vi "State_Machine.vi"(8 "error in (no error)":errorcluster caption="entrée d'erreur (pas d'erreur)", 11 "Get_Voltage en entrée":refnum<class "Zigbee_Send_Msg_Default.lvclass">) -> (0 "error out":errorcluster caption="sortie d'erreur", 2 "Json_String":string, 3 "Get_Voltage en sortie":refnum<class "Zigbee_Send_Msg_Default.lvclass">)   [LabVIEW 2020, in "Library Test.lvlib" / "Zigbee_Send_Msg_Default.lvclass"]
uses:
  Zigbee_Send_Msg_Default.lvclass
  C:/Users/ngarcin/OneDrive - Altyor/Standard TB/Class/Test/Zigbee_Send_Msg/Zigbee_Send_Msg.lvclass
  Zigbee_Send_Msg/Zigbee_Send_Msg.lvclass
  Zigbee_Send_Msg_Default.lvclass/Zigbee_Send_Msg_Default.ctl
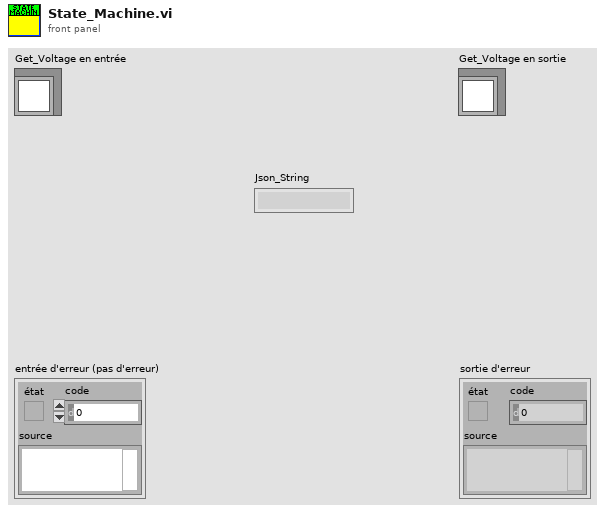
[diagram p1: front panel]
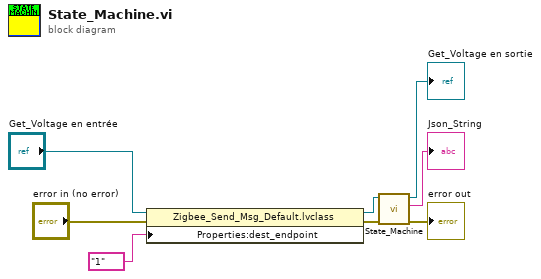
[diagram p0: block diagram]
diagram:
  n1 = property class="Zigbee_Send_Msg_Default.lvclass"(reference="Get_Voltage en entrée", error in="error in (no error)", "Properties:dest_endpoint"="1") -> (reference out=w4:refnum<class "Zigbee_Send_Msg_Default.lvclass">, error out=w1:errorcluster)
  n2 = call-parent "State_Machine.vi"("error in (no error)"=w1, "Get_Voltage en entrée"=w4) -> ("error out"=→"error out":errorcluster, "Json_String"=→"Json_String":string, "Get_Voltage en sortie"=→"Get_Voltage en sortie":refnum<class "Zigbee_Send_Msg_Default.lvclass">)  [unwired: 7 in]
